vi "subFile Dialog.vi"(0 "start path":path, 1 "prompt":string, 3 "button label":string, 5 "selection mode":T1(ring), 7 "default name":string, 11 "error in":errorcluster, 12 "pattern (all files)":string, 14 "pattern label":string) -> (4 "selected path":path, 6 "selected paths":path[](array[path]), 8 "exists":bool, 10 "cancelled":bool, 15 "error out":errorcluster)   [LabVIEW 2010]
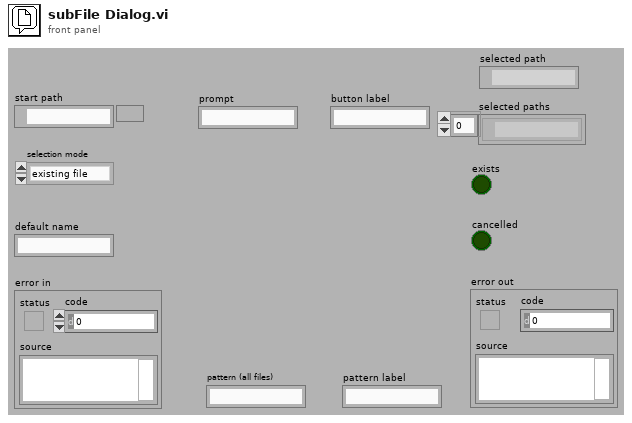
[diagram p1: front panel]
types:
  T1 = enum32{"existing file", "new file", "new or existing file", "existing dir", "new dir", "new or existing dir", "existing file (use LLBs)", "new file (use LLBs)", "new or existing file (use LLBs)", "new or existing file or directory (use LLBs)", "existing dir (use LLBs)", "new dir (use LLBs)", "new or existing dir (use LLBs)", "existing file or dir", "new file or dir", "new or existing file or dir", "existing file or dir (use LLBs)", "new file or dir (use LLBs)", "multi-select", "multi-select (use LLBs)"}
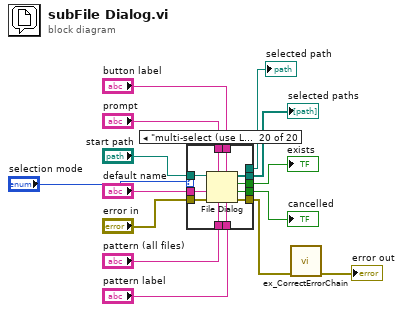
[diagram p0: block diagram]
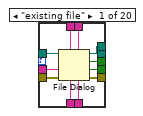
[diagram p2: hidden frame]
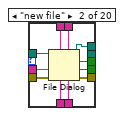
[diagram p3: hidden frame]
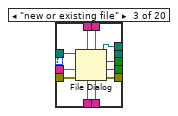
[diagram p4: hidden frame]
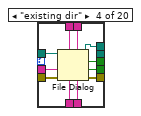
[diagram p5: hidden frame]
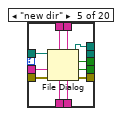
[diagram p6: hidden frame]
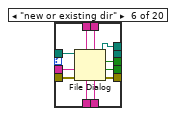
[diagram p7: hidden frame]
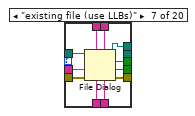
[diagram p8: hidden frame]
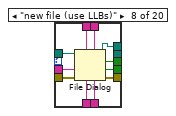
[diagram p9: hidden frame]
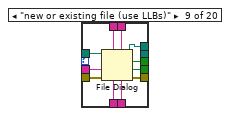
[diagram p10: hidden frame]
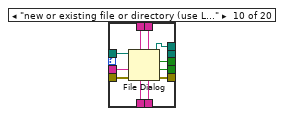
[diagram p11: hidden frame]
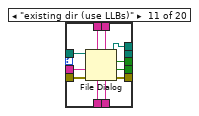
[diagram p12: hidden frame]
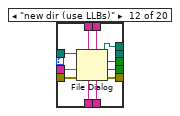
[diagram p13: hidden frame]
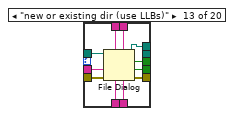
[diagram p14: hidden frame]
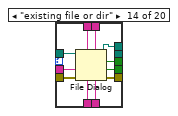
[diagram p15: hidden frame]
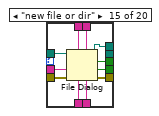
[diagram p16: hidden frame]
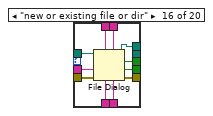
[diagram p17: hidden frame]
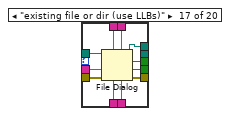
[diagram p18: hidden frame]
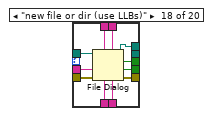
[diagram p19: hidden frame]
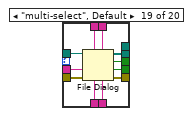
[diagram p20: hidden frame]
diagram:
  n1 = case shown="\"multi-select (use LLBs)\"" "selection mode" {
    tunnel: "start path" -> [w25 w36 w47 w58 w69 w80 w91 w102 w113 w124 w135 w146 w157 w168 w179 w190 w201 w212 w223 w234]
    tunnel: "default name" -> [w24 w35 w46 w57 w68 w79 w90 w101 w112 w123 w134 w145 w156 w167 w178 w189 w200 w211 w222 w233]
    tunnel: "error in" -> [w23 w34 w45 w56 w67 w78 w89 w100 w111 w122 w133 w144 w155 w166 w177 w188 w199 w210 w221 w232]
    tunnel: "pattern (all files)" -> [w22 w33 w44 w55 w66 w77 w88 w99 w110 w121 w132 w143 w154 w165 w176 w187 w198 w209 w220 w231]
    tunnel: "prompt" -> [w21 w32 w43 w54 w65 w76 w87 w98 w109 w120 w131 w142 w153 w164 w175 w186 w197 w208 w219 w230]
    tunnel: "button label" -> [w20 w31 w42 w53 w64 w75 w86 w97 w108 w119 w130 w141 w152 w163 w174 w185 w196 w207 w218 w229]
    tunnel: "pattern label" -> [w19 w30 w41 w52 w63 w74 w85 w96 w107 w118 w129 w140 w151 w162 w173 w184 w195 w206 w217 w228]
    tunnel: [_ _ _ _ _ _ _ _ _ _ _ _ _ _ _ _ _ _ w213 w224] -> w5
    tunnel: [w18 w29 w40 w51 w62 w73 w84 w95 w106 w117 w128 w139 w150 w161 w172 w183 w194 w205 w216 w227] -> w7
    tunnel: [w17 w28 w39 w50 w61 w72 w83 w94 w105 w116 w127 w138 w149 w160 w171 w182 w193 w204 w215 w226] -> w6
    tunnel: [w16 w27 w38 w49 w60 w71 w82 w93 w104 w115 w126 w137 w148 w159 w170 w181 w192 w203 w214 w225] -> w2
    tunnel: [w15 w26 w37 w48 w59 w70 w81 w92 w103 w114 w125 w136 w147 w158 w169 w180 w191 w202 _ _] -> w4
    frame "existing file" {
      n2 = File Dialog(4:w19, 5:w20, 6:w22, 7:w21, 8:w23, 9:w24, 11:w25) -> (0:w16:errorcluster, 1:w17:bool, 2:w18:bool, 3:w15:path)
    }
    frame "new file" {
      n3 = File Dialog(4:w30, 5:w31, 6:w33, 7:w32, 8:w34, 9:w35, 11:w36) -> (0:w27:errorcluster, 1:w28:bool, 2:w29:bool, 3:w26:path)
    }
    frame "new or existing file" {
      n4 = File Dialog(4:w41, 5:w42, 6:w44, 7:w43, 8:w45, 9:w46, 11:w47) -> (0:w38:errorcluster, 1:w39:bool, 2:w40:bool, 3:w37:path)
    }
    frame "existing dir" {
      n5 = File Dialog(4:w52, 5:w53, 6:w55, 7:w54, 8:w56, 9:w57, 11:w58) -> (0:w49:errorcluster, 1:w50:bool, 2:w51:bool, 3:w48:path)
    }
    frame "new dir" {
      n6 = File Dialog(4:w63, 5:w64, 6:w66, 7:w65, 8:w67, 9:w68, 11:w69) -> (0:w60:errorcluster, 1:w61:bool, 2:w62:bool, 3:w59:path)
    }
    frame "new or existing dir" {
      n7 = File Dialog(4:w74, 5:w75, 6:w77, 7:w76, 8:w78, 9:w79, 11:w80) -> (0:w71:errorcluster, 1:w72:bool, 2:w73:bool, 3:w70:path)
    }
    frame "existing file (use LLBs)" {
      n8 = File Dialog(4:w85, 5:w86, 6:w88, 7:w87, 8:w89, 9:w90, 11:w91) -> (0:w82:errorcluster, 1:w83:bool, 2:w84:bool, 3:w81:path)
    }
    frame "new file (use LLBs)" {
      n9 = File Dialog(4:w96, 5:w97, 6:w99, 7:w98, 8:w100, 9:w101, 11:w102) -> (0:w93:errorcluster, 1:w94:bool, 2:w95:bool, 3:w92:path)
    }
    frame "new or existing file (use LLBs)" {
      n10 = File Dialog(4:w107, 5:w108, 6:w110, 7:w109, 8:w111, 9:w112, 11:w113) -> (0:w104:errorcluster, 1:w105:bool, 2:w106:bool, 3:w103:path)
    }
    frame "new or existing file or directory (use LLBs)" {
      n11 = File Dialog(4:w118, 5:w119, 6:w121, 7:w120, 8:w122, 9:w123, 11:w124) -> (0:w115:errorcluster, 1:w116:bool, 2:w117:bool, 3:w114:path)
    }
    frame "existing dir (use LLBs)" {
      n12 = File Dialog(4:w129, 5:w130, 6:w132, 7:w131, 8:w133, 9:w134, 11:w135) -> (0:w126:errorcluster, 1:w127:bool, 2:w128:bool, 3:w125:path)
    }
    frame "new dir (use LLBs)" {
      n13 = File Dialog(4:w140, 5:w141, 6:w143, 7:w142, 8:w144, 9:w145, 11:w146) -> (0:w137:errorcluster, 1:w138:bool, 2:w139:bool, 3:w136:path)
    }
    frame "new or existing dir (use LLBs)" {
      n14 = File Dialog(4:w151, 5:w152, 6:w154, 7:w153, 8:w155, 9:w156, 11:w157) -> (0:w148:errorcluster, 1:w149:bool, 2:w150:bool, 3:w147:path)
    }
    frame "existing file or dir" {
      n15 = File Dialog(4:w162, 5:w163, 6:w165, 7:w164, 8:w166, 9:w167, 11:w168) -> (0:w159:errorcluster, 1:w160:bool, 2:w161:bool, 3:w158:path)
    }
    frame "new file or dir" {
      n16 = File Dialog(4:w173, 5:w174, 6:w176, 7:w175, 8:w177, 9:w178, 11:w179) -> (0:w170:errorcluster, 1:w171:bool, 2:w172:bool, 3:w169:path)
    }
    frame "new or existing file or dir" {
      n17 = File Dialog(4:w184, 5:w185, 6:w187, 7:w186, 8:w188, 9:w189, 11:w190) -> (0:w181:errorcluster, 1:w182:bool, 2:w183:bool, 3:w180:path)
    }
    frame "existing file or dir (use LLBs)" {
      n18 = File Dialog(4:w195, 5:w196, 6:w198, 7:w197, 8:w199, 9:w200, 11:w201) -> (0:w192:errorcluster, 1:w193:bool, 2:w194:bool, 3:w191:path)
    }
    frame "new file or dir (use LLBs)" {
      n19 = File Dialog(4:w206, 5:w207, 6:w209, 7:w208, 8:w210, 9:w211, 11:w212) -> (0:w203:errorcluster, 1:w204:bool, 2:w205:bool, 3:w202:path)
    }
    frame "multi-select", Default {
      n20 = File Dialog(4:w217, 5:w218, 6:w220, 7:w219, 8:w221, 9:w222, 11:w223) -> (0:w214:errorcluster, 1:w215:bool, 2:w216:bool, 3:w213:path[])
    }
    frame "multi-select (use LLBs)" {
      n21 = File Dialog(4:w228, 5:w229, 6:w231, 7:w230, 8:w232, 9:w233, 11:w234) -> (0:w225:errorcluster, 1:w226:bool, 2:w227:bool, 3:w224:path[])
    }
  }
  "exists" <- w7
  "cancelled" <- w6
  "selected paths" <- w5
  "selected path" <- w4
  n22 = call "ex_CorrectErrorChain.vi"("error in (no error)"=w2) -> ("error out"=→"error out":errorcluster)  [unwired: 10 in]
